vi "Test Metric.vi"() -> ()   [LabVIEW 2020]
uses:
  src/metrics/counter/Counter.lvclass
  src/registry/session/Registry Session.lvclass
  src/metrics/histogram/Histogram.lvclass
panel:
  out "Next Timeout":i32
  out "Metric Names":string[](array[string])
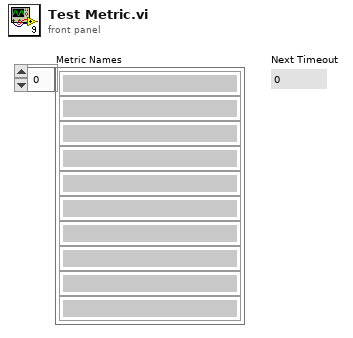
[diagram p1: front panel]
types:
  T1 = typedef "Registry.lvlib/Registry Session.lvclass/Session Handle.ctl" = refnum<data-value>
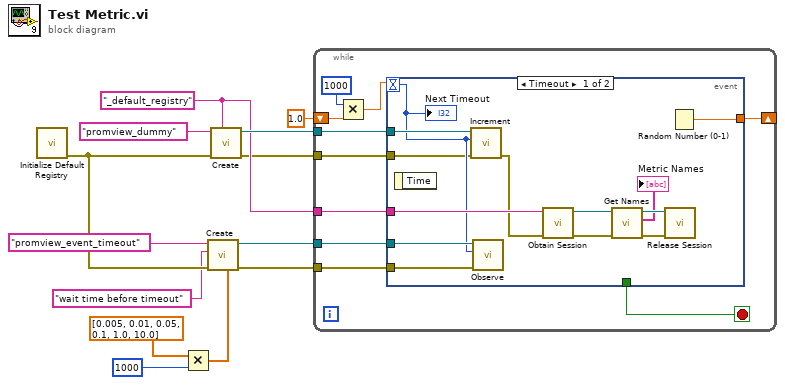
[diagram p0: block diagram]
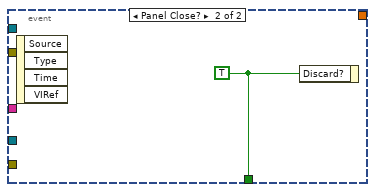
[diagram p2: hidden frame]
diagram:
  w11 = "_default_registry" ("Registry Name")
  n1 = call "Initialize Default Registry.vi"() -> ("error out"=w9:errorcluster)  [unwired: 9 in, 2 out]
  n2 = Multiply(x=dbl[] [0.005, 0.01, 0.05, 0.1, 1.0, 10.0] ("Buckets"), y=1000) -> (x*y=w5:dbl[])
  n3 = call "Create.vi"("Buckets"=w5, "error in (no error)"=w9, "Description"="wait time before timeout", "Name"="promview_event_timeout") -> ("error out"=w4:errorcluster, "Histogram Ref"=w6:refnum<data-value>)  [unwired: 6 in]
  n4 = call "Create.vi"("Registry Name"=w11, "error in (no error)"=w9, "Metric Name"="promview_dummy") -> ("error out"=w3:errorcluster, "Counter Ref"=w13:refnum<data-value>)  [unwired: 7 in]
  n5 = while {
    tunnel: w13 -> [w22]
    tunnel: w11 -> [w21]
    shift-right: [w19] -> _
    shift-left: 1.0 ("number: 0 to 1") -> [w18]
    tunnel: w6 -> [w16]
    tunnel: w4 -> [w15]
    tunnel: w3 -> [w14]
    stop <- w23 stop-if-true
    n6 = Multiply(x=1000, y=w18) -> (x*y=w17:dbl)
    n7 = event shown="[0] Timeout" {
      selector: _ -> [_ _]
      dyn-events: _ -> [_ _]
      timeout: w17 -> [w28 _]
      tunnel: [_ w37] -> w23
      tunnel: w22 -> [w36 _]
      tunnel: w21 -> [w35 _]
      tunnel: [w30 _] -> w19
      tunnel: w16 -> [w29 _]
      tunnel: w15 -> [w27 _]
      tunnel: w14 -> [w26 _]
      event Timeout {
        n8 = event-data() -> ()  [unwired: 1 in, 1 out]
        n9 = call "Increment.vi"("error in (no error)"=w26, "Step"=w28, "Counter Ref"=w36) -> ("error out"=w34:errorcluster)  [unwired: 7 in, 1 out]
        n10 = call "Observe.vi"("error in (no error)"=w27, "New Value"=w28, "Histogram Ref"=w29) -> ()  [unwired: 7 in, 2 out]
        n11 = call "Obtain Session.vi"("error in (no error)"=w34, "Session  Name ()"=w35) -> ("error out"=w25:errorcluster, "Session Handle"=w31:T1)  [unwired: 8 in]
        n12 = call "Get Names.vi"("error in (no error)"=w25, "Session Handle in"=w31) -> ("error out"=w24:errorcluster, "Metric Names"=→"Metric Names":string[], "Session Handle out"=w33:T1)  [unwired: 7 in]
        n13 = call "Release Session.vi"("error in (no error)"=w24, "Session Handle"=w33) -> ()  [unwired: 9 in, 1 out]
        n14 = Random Number (0-1)() -> (number: 0 to 1=w30:dbl)
        "Next Timeout" <- w28
      }
      event Panel Close? {
        w37 = TRUE ("Discard?")
        n15 = event-data() -> ()  [unwired: 1 in, 4 out]
        n16 = event-data("Discard?"=w37) -> ()  [unwired: 1 in, 1 out]
      }
    }
  }
